vi "Task.vi"(8 "error in (no error)":errorcluster, 10 "Data":i32, 11 "HAL Interface Actor in":refnum<class "HAL Interface Actor.lvclass">) -> (0 "error out":errorcluster, 3 "HAL Interface Actor out":refnum<class "HAL Interface Actor.lvclass">)   [LabVIEW 2024, in "HAL Interface Actor.lvlib" / "HAL Interface Actor.lvclass"]
uses:
  HAL Interface Actor.lvclass
  C:/Program Files (x86)/National Instruments/LabVIEW 2024/vi.lib/ActorFramework/Actor/Actor.lvclass
  <vilib>/ActorFramework/Actor/Actor.lvclass/Actor.ctl
  App Actor/Log Event Msg/Log Event Msg.lvclass/Log Event Msg.ctl
  <vilib>/ActorFramework/Message Enqueuer/Message Enqueuer.lvclass/Message Enqueuer.ctl
  <vilib>/ActorFramework/Message Enqueuer/Enqueue.vi
  App Actor/Log Event Msg/Log Event Msg.lvclass
  C:/Program Files (x86)/National Instruments/LabVIEW 2024/vi.lib/ActorFramework/Message/Message.lvclass
  <vilib>/ActorFramework/Message Priority Queue/Priority Enqueue.vi
  <vilib>/ActorFramework/Actor/Actor.lvclass
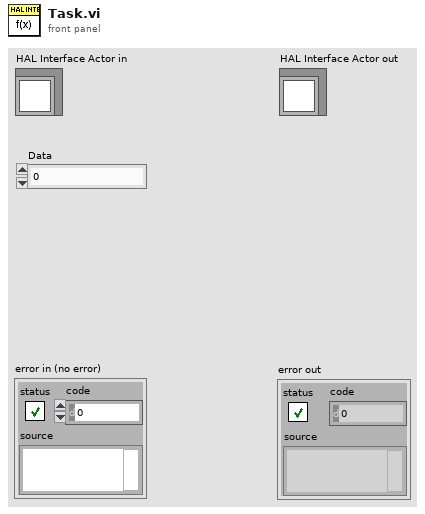
[diagram p1: front panel]
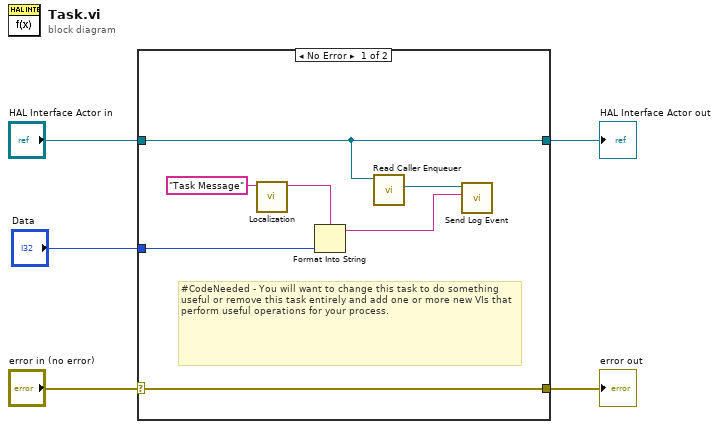
[diagram p0: block diagram]
diagram:
  n1 = case shown="No Error" "error in (no error)" {
    selector: "error in (no error)" -> [w12 w14]
    tunnel: [w12 w14] -> w4
    tunnel: [w11 w13] -> w2
    tunnel: "HAL Interface Actor in" -> [w11 w13]
    tunnel: "Data" -> [w7 _]
    frame No Error {
      # "#CodeNeeded - You will want to change this task to do something useful or remove this task entirely and add one or more new VIs that perform useful operations for your process."
      n2 = call "Localization.vi"("Unlocalized"="Task Message") -> ("Localized"=w8:string)  [unwired: 10 in]
      n3 = Format Into String(format string=w8, w7) -> (resulting string=w6:string)  [unwired: 2 in, 1 out]
      n4 = call <vilib>:"Read Caller Enqueuer.vi"("Actor"=w11) -> ("Caller Enqueuer"=w10:refnum<class "Message Enqueuer.lvclass">)  [unwired: 10 in]
      n5 = call "Send Log Event.vi"("Event Text"=w6, "Message Enqueuer"=w10) -> ()  [unwired: 9 in, 1 out]
    }
    frame Error {
    }
  }
  "error out" <- w4
  "HAL Interface Actor out" <- w2
